vi "init.vi"(8 "error in (no error)":errorcluster, 10 "Init Data":variant, 11 "Lakeshore 331 in":refnum<class "Lakeshore 331.lvclass">) -> (0 "error out":errorcluster, 2 "Channel List":refnum<class "HK Item.lvclass">[](array[class]), 3 "Lakeshore 331 out":refnum<class "Lakeshore 331.lvclass">)   [LabVIEW 2022 SP3, in "Lakeshore 331.lvclass"]
uses:
  Lakeshore 331.lvclass
  hk-channel-class/hk-channel-class/HK Item/HK Item.lvclass
  Lakeshore 331.lvclass/Lakeshore 331.ctl
  <instrlib>/Lake Shore Cryotronics 331/Lake Shore Cryotronics 331.lvlib
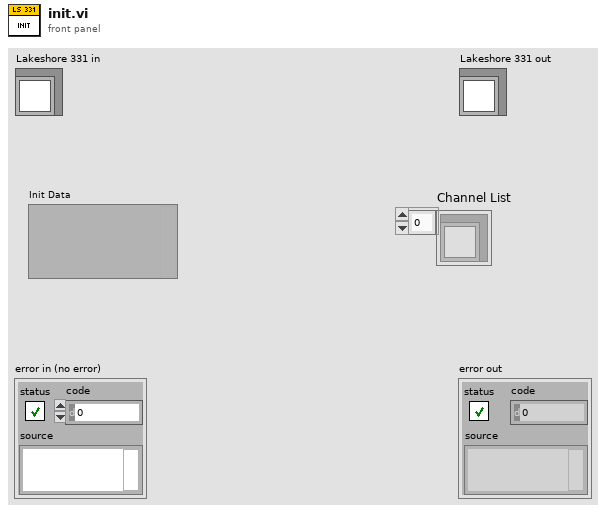
[diagram p1: front panel]
types:
  T1 = typedef "Lakeshore 331.lvclass/Lakeshore 331 Settings.ctl" = cluster{"Addr":refnum<visa-resource-name>, "Ch Prefix":string, "Ch Select":i32[]}
  T2 = typedef "Temp Control.lvclass/Temp Control Parameters.ctl" = cluster{"Mode":u16, "Setpoint":dbl, "Manual Power (%)":dbl, "Control Parameters":cluster{"P":dbl, "I":dbl, "D":u16}, "Heater Range":u16, "Default Range":u16}
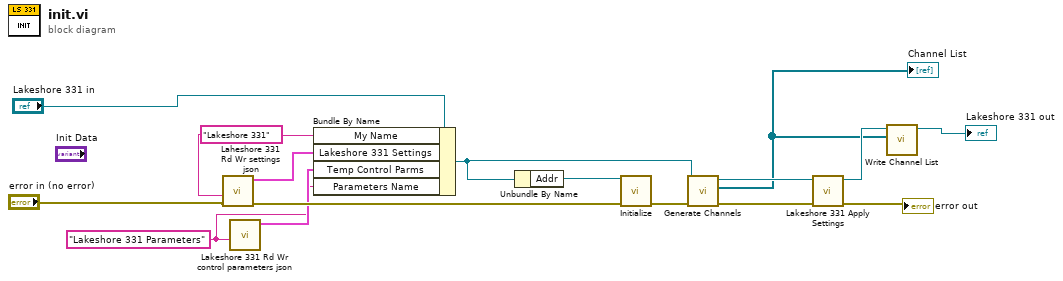
[diagram p0: block diagram]
diagram:
  w11 = "Lakeshore 331 Parameters" ("section")
  w13 = "Lakeshore 331" ("section")
  n1 = call "Laheshore 331 Rd Wr settings json.vi"("error in (no error)"="error in (no error)", "section"=w13) -> ("error out"=w14:errorcluster, "Lakeshore 331 Settings"=w15:T1)  [unwired: 8 in]
  n2 = call "Lakeshore 331 Rd Wr control parameters json.vi"("Section"=w11) -> ("Temp Control Parms"=w12:T2)  [unwired: 9 in, 1 out]
  n3 = Bundle By Name(cluster="Lakeshore 331 in", "My Name"=w13, "Lakeshore 331 Settings"=w15, "Temp Control Parms"=w12, "Parameters Name"=w11) -> (w10:refnum<class "Lakeshore 331.lvclass">)
  n4 = Unbundle By Name(w10) -> ("Addr"=w16:refnum<visa-resource-name>)
  n5 = call <instrlib>:"Initialize.vi"("VISA resource name"=w16, "error in (no error)"=w14) -> ("error out"=w6:errorcluster)  [unwired: 12 in, 1 out]
  n6 = call-dynamic "Generate Channels.vi"("error in (no error)"=w6, "Lakeshore 331 in"=w10) -> ("error out"=w7:errorcluster, "Channel List"=w1:refnum<class "HK Item.lvclass">[], "Lakeshore 331 out"=w5:refnum<class "Lakeshore 331.lvclass">)  [unwired: 6 in, 1 out]
  "Channel List" <- w1
  n7 = call "Lakeshore 331 Apply Settings.vi"("error in (no error)"=w7, "Lakeshore 331 in"=w5) -> ("error out"=→"error out":errorcluster, "Lakeshore 331 out"=w3:refnum<class "Lakeshore 331.lvclass">)  [unwired: 8 in]
  n8 = call-dynamic "Write Channel List.vi"("Channel List"=w1, "Temp Control in"=w3) -> ("Temp Control out"=→"Lakeshore 331 out":refnum<class "Lakeshore 331.lvclass">)  [unwired: 8 in, 1 out]
